vi "set_crystal_speed.vi"(8 "error in":errorcluster, 9 "Crystal Speed / counts s-1":dbl, 10 "Crystal Number":u16(ring) items=["Crystal 1", "Crystal 2", "Crystal 3", "Crystal 4", "Crystal 5", "Crystal 6", "Crystal 7", ""], 11 "address":string) -> (0 "error out":errorcluster, 2 "Crystal Number Out":u16(ring) items=["Crystal 1", "Crystal 2", "Crystal 3", "Crystal 4", "Crystal 5", "Crystal 6", "Crystal 7", ""])   [LabVIEW 2020]
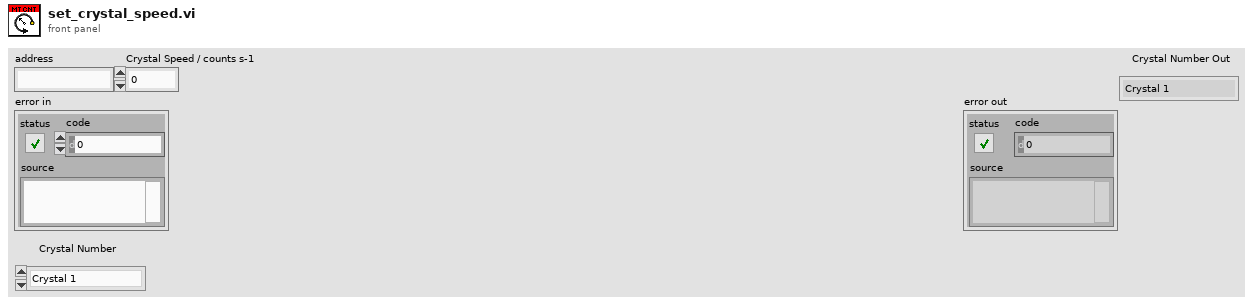
[diagram p1: front panel]
types:
  T1 = enum16{"Standard", "Buffered", "CRLF", "Immediate"}
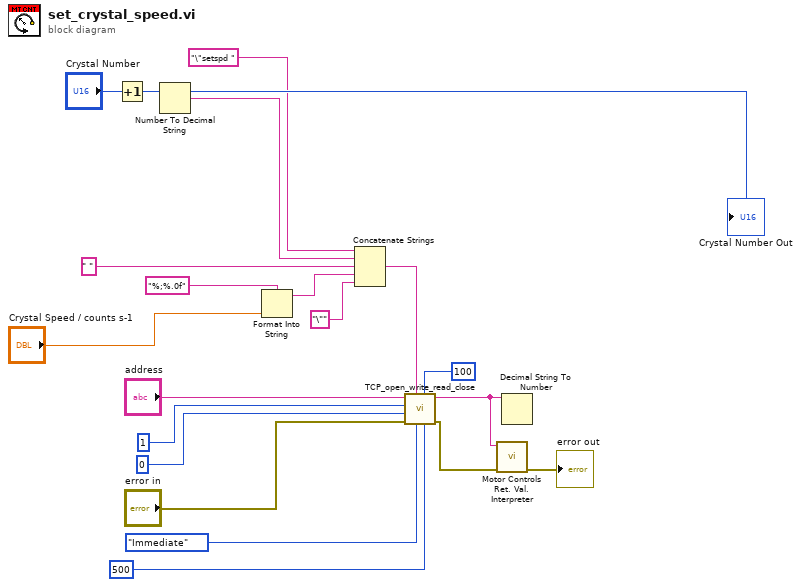
[diagram p0: block diagram]
diagram:
  n1 = Increment(x="Crystal Number") -> (x+1=w19:u16)
  n2 = Number To Decimal String(number=w19) -> (decimal integer string=w12:string)  [unwired: 1 in]
  n3 = Format Into String(format string="%;%.0f", "Crystal Speed / counts s-1") -> (resulting string=w5:string)  [unwired: 2 in, 1 out]
  n4 = Concatenate Strings("\"setspd " ("write string"), w12, " " ("string"), w5, "\"" ("string")) -> (w11:string)
  n5 = call "TCP_open_write_read_close.vi"("timeout ms (25000)"=500, "bytes to read"=100, "mode (standard)"=T1."Immediate", "write string"=w11, "error in"="error in", "local port (0)"=u16 0, "remote port or service name"=u16 1, "address"="address") -> ("error out"=w9:errorcluster, "read string"=w7:string)  [unwired: 2 in]
  n6 = call "Motor Controls Ret. Val. Interpreter.vi"("error in"=w9, "Command Return"=w7) -> ("error out"=→"error out":errorcluster)  [unwired: 8 in, 1 out]
  n7 = Decimal String To Number(string=w7) -> ()  [unwired: 2 in, 2 out]
  "Crystal Number Out" <- "Crystal Number"
